vi "GUI Update Range Selectors.vi"(1 "total channels":i32, 2 "range mode":T1 caption="Voltage range selection", 3 "odd and even item names":string) -> (0 "ranges vector [V]":dbl[](array[numeric]))   [LabVIEW 2013]
doc: "Updates controls for voltage range selection using SGUI lib. Enter names of the Odd and Even range control as multiline string."
uses:
  Meas Range Mode.ctl
  varilib/varilib.lvlib
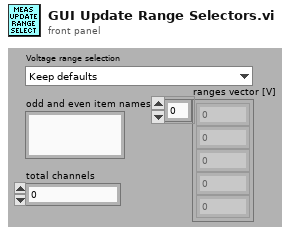
[diagram p1: front panel]
types:
  T1 = typedef "Meas Range Mode.ctl" = enum16{"Keep defaults", "Set All channels", "Set Odd and Even channels"}
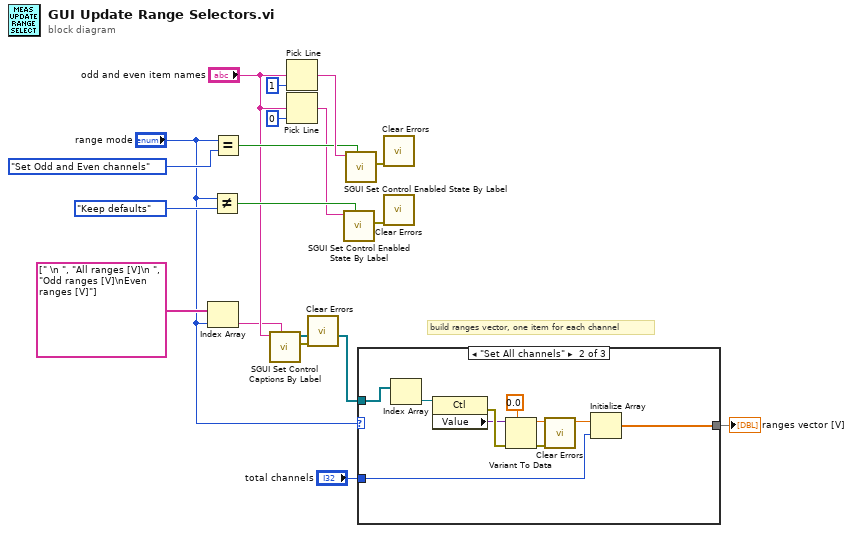
[diagram p0: block diagram]
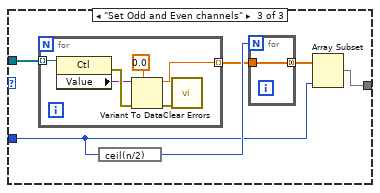
[diagram p3: hidden frame]
diagram:
  # "build ranges vector, one item for each channel"
  n1 = Index Array(array=string[] [" \n ", "All ranges [V]\n ", "Odd ranges [V]\nEven ranges [V]"], index="range mode") -> (element=w8:string)
  n2 = Not Equal?(x="range mode", y=Meas_Range_Mode."Keep defaults") -> (x != y?=w12:bool)
  n3 = Equal?(x="range mode", y=Meas_Range_Mode."Set Odd and Even channels") -> (x = y?=w13:bool)
  n4 = call "SGUI Set Control Captions By Label.vi"("labels (empty)"="odd and even item names", "captions (empty)"=w8) -> ("error out"=w2:errorcluster, "control references out"=w6:refnum<vi>[])  [unwired: 8 in]
  n5 = Pick Line(multi-line string="odd and even item names", line index=1) -> (output string=w14:string)  [unwired: 1 in]
  n6 = Pick Line(multi-line string="odd and even item names", line index=0) -> (output string=w11:string)  [unwired: 1 in]
  n7 = call <vilib>:"Clear Errors.vi"("error in (no error)"=w2) -> ()  [unwired: 6 in, 1 out]
  n8 = call "SGUI Set Control Enabled State By Label.vi"("labels (empty)"=w11, "Enabled? (False)"=w12) -> ("error out"=w3:errorcluster)  [unwired: 8 in, 1 out]
  n9 = call "SGUI Set Control Enabled State By Label.vi"("labels (empty)"=w14, "Enabled? (False)"=w13) -> ("error out"=w4:errorcluster)  [unwired: 8 in, 1 out]
  n10 = case shown="\"Set All channels\"" "range mode" {
    tunnel: w6 -> [_ w26 w33]
    tunnel: "total channels" -> [_ w21 w29]
    tunnel: [_ w20 w28] -> w1
    frame Default {
    }
    frame "Set All channels" {
      n11 = Index Array(array=w26) -> (element=w27:refnum<vi>)  [unwired: 1 in]
      n12 = property class="Ctl"(reference=w27) -> (error out=w25:errorcluster, "Value"=w24:variant)  [unwired: 1 in, 1 out]
      n13 = Variant To Data(error in=w25, type=0.0, Variant=w24) -> (data=w22:dbl, error out=w19:errorcluster)
      n14 = call <vilib>:"Clear Errors.vi"("error in (no error)"=w19) -> ()  [unwired: 6 in, 1 out]
      n15 = Initialize Array(w22, w21) -> (w20:dbl[])
    }
    frame "Set Odd and Even channels" {
      n16 = for {
        tunnel: w33 -> [w37] mode=indexing
        tunnel: [w35] -> w31 mode=indexing
        n17 = property class="Ctl"(reference=w37) -> (error out=w40:errorcluster, "Value"=w39:variant)  [unwired: 1 in, 1 out]
        n18 = Variant To Data(error in=w40, type=0.0, Variant=w39) -> (data=w35:dbl, error out=w36:errorcluster)
        n19 = call <vilib>:"Clear Errors.vi"("error in (no error)"=w36) -> ()  [unwired: 6 in, 1 out]
      }
      n20 = expression code="ceil(n/2)"(w29) -> (w32:i32)
      n21 = for {
        N: w32 -> [_]
        tunnel: w31 -> [w34]
        tunnel: [w34] -> w30 mode=concatenating
      }
      n22 = Array Subset(array=w30, length=w29) -> (w28:dbl[])  [unwired: 1 in]
    }
  }
  "ranges vector [V]" <- w1
  n23 = call <vilib>:"Clear Errors.vi"("error in (no error)"=w4) -> ()  [unwired: 6 in, 1 out]
  n24 = call <vilib>:"Clear Errors.vi"("error in (no error)"=w3) -> ()  [unwired: 6 in, 1 out]
